vi "二维动态避障简单测试0502(4070双远程版).vi"() -> ()   [LabVIEW 2018]
doc: "Demonstrates the use of the Network Streams functions to send LED status to the myRIO target."
uses:
  <vilib>/addons/zeromq/socket_type.ctl
  <vilib>/ErrorRing/Error Ring.xnode
  <vilib>/vision/NI_Vision_Development_Module.lvlib
  <vilib>/addons/zeromq/zmq_socket.lvclass
  <vilib>/addons/zeromq/zmq_context.lvclass
  <vilib>/addons/zeromq/zeromq.lvlib
panel:
  out "c2":ext
  out "c1":ext
  out "next_relative_desired_point_y":ext
  out "next_relative_desired_point_x":ext
  in  "簇 14":cluster{"c1":ext, "c2":ext}={"c1"=100000.0, "c2"=100000.0}
  out "relative_real_y_color 2":dbl=2.0
  out "relative_real_x_color 2":dbl=2.0
  in  "簇 13":T1={"relative_real_x_color"=100000.0, "relative_real_y_color"=1.0, "t"=1.0}
  out "u(t)_y":ext
  out "u(t)_x":ext
  out "relative_real_y_color":ext
  out "relative_real_x_color":ext
  in  "中心轨迹":bool
  in  "打开彩色点轨迹":bool
  out "relative_real_y_color":ext
  out "relative_real_x_color":ext
  out "彩色轨迹":T2(plugin-control)
  out "end_point_y":ext
  out "end_point_x":ext
  out "cy":ext
  out "cx":ext
  out "c":ext
  in  "簇 10":T3={"c"=100000.0, "cx"=100000.0, "cy"=100000.0, "start_point_x"=100000.0, "start_point_y"=100000.0}
  out "输出簇":T4
  in  "簇 9":T4={"a"=[], "b"=1.0, "a2"=[], "left1"=1.0, "top1"=1.0, "left2"=1.0, "top2"=1.0, "delta1"=1.0, "delta2"=1.0}
  in  "delta2":dbl=130.0
  out "bottom2":dbl
  out "right2":dbl
  out "top2":dbl
  out "left2":dbl
  in  "delta1":dbl=130.0
  out "bottom1":dbl
  out "right1":dbl
  out "top1":dbl
  out "left1":dbl
  out "delta_pr":dbl
  out "delta_dr":dbl
  in  "k2":dbl=-0.3
  in  "K1":dbl=0.3
  in  "Operation":T5(ring)=enum."Erode"
  out "old_real_relative_point_y":dbl
  out "old_real_relative_point_x":dbl
  out "real_relative_start_point_y":dbl
  out "real_relative_start_point_x":dbl
  out "Bounding Box.Y Top 2":i32
  out "Bounding Box.X Left 2":i32
  out "Ki part":dbl
  out "Kd part":dbl
  out "Kp part":dbl
  out "Ki part":dbl
  out "Kd part":dbl
  out "Kp part":dbl
  in  "Ki":dbl=0.004
  in  "Kd":dbl=1e-05
  in  "Kp":dbl=0.013
  in  "Ki":dbl=0.0035
  in  "Kd":dbl=1e-05
  in  "Kp":dbl=0.013
  out "添加的数组":dbl[](array[numeric])
  out "desired_relative_point_y":dbl=820.0
  out "desired_relative_point_x":dbl=730.0
  out "MLP_pr":dbl=20.0
  out "MLP_dr":dbl=8.0
  out "error_relative_point_y":dbl
  out "error_relative_point_x":dbl
  out "real_relative_end_point_y":dbl
  out "real_relative_end_point_x":dbl
  out "magnet_input_pr":dbl
  out "magnet_input_dr":dbl
  in  "打开仅尖端轨迹":bool
  out "仅尖端轨迹":T2(plugin-control)
  out "Bounding Box.Y Top":i32
  out "Bounding Box.X Left":i32
  out "curve_min_y":dbl
  out "curve_min_x":dbl
  out "curve_max_y":dbl
  out "curve_max_x":dbl
  out "relative_end_point_y":dbl
  out "relative_end_point_x":dbl
  out "delta_y":dbl
  out "delta_x":dbl
  out "pr":dbl=-28.0
  out "tan(v)":dbl
  out "delta_velocity":dbl format="%#_10g"
  out "delta_time":dbl
  out "now time":timestamp[](array[timestamp])
  out "prev time":timestamp[](array[timestamp])
  out "delta_distance":dbl
  out "prev_end_point_y":dbl
  out "prev_end_point_x":dbl
  out "now_end_point_y":dbl
  out "now_end_point_x":dbl
  out "prev_end_point_y":dbl[](array[numeric])
  out "prev_end_point_x":dbl[](array[numeric])
  out "dr":dbl=120.0
  in  "Ar":sgl=11.0
  out "all parameters":dbl[][](array[numeric])
  out "direction angle":sgl[](array[numeric])
  out "dr":sgl
  out "strength":dbl[](array[numeric])
  out "场强":dbl
  out "end_point_y":T6
  out "end_point_x":dbl[](array[numeric])
  out "start_point_y":dbl[](array[numeric])
  out "start_point_x":dbl[](array[numeric])
  out "T":i32[](array[numeric])
  out "c":dbl[](array[numeric])
  out "b":dbl[](array[numeric])
  out "a\na":dbl[](array[numeric])
  out "c":dbl
  out "b":dbl
  out "a":dbl
  out "Angles (deg)":sgl[](array[numeric]) format="%.2f"
  in  "wr":sgl
  in  "打开轨迹":bool
  out "中心轨迹和尖端轨迹":T2(plugin-control)
  out "end_y":dbl
  out "end_x":dbl
  out "start_y":dbl
  out "start_x":dbl
  out "Image Pixels (U8)":u8[][](array[numeric])
  in  "Poly":dbl
  out "中心轨迹":T2(plugin-control)
  in  "保存按钮":bool
  out "Object Center":cluster{"X":sgl, "Y":sgl}
  out "黑白图":T2(plugin-control)
  in  "Number of Erosion":i32=5
  in  "Settings":T7={"Objects"=1, "Threshold"=128, "Reject Border"=FALSE, "Fill Holes"=FALSE, "Min Object Size"=TRUE, "Min Size"=1200, "Max Object Size"=FALSE, "Max Size"=100, "Show Search Area"=TRUE, "Show Center"=TRUE, "Show Bounding Box"=TRUE} {"Objects" items=["Bright Objects", "Dark Objects"]; "Threshold" min=1 max=999999999 step=1; "Max Size" min=1 max=999999999 step=1; "Min Size" min=1 max=999999999 step=1}
  out "Objects":T8(array[cluster]) {"Aspect Ratio" format="%.2f"; "Orientation" format="%.2f"; "Area" format="%.2f"; "Object Center"."Y" format="%.2f"; "Object Center"."X" format="%.2f"}
  in  "Search Rect (entire image)":T9={"Left"=350, "Top"=100, "Right"=1020, "Bottom"=1030, "Rotation"=0.0} {"Rotation" format="%.2f"; "Left" scale=0.0..1024.0; "Right" scale=0.0..1024.0}
  in  "Range":cluster{"Lower value":sgl, "Upper value":sgl}={"Lower value"=177.0, "Upper value"=255.0} {"Upper value" format="%.2f"; "Lower value" format="%.2f"}
  out "原图":T2(plugin-control)
  in  "停止":bool
  out "T":i32
  out "T":i32
  in  "磁场变换":bool=TRUE
  in  "Pause":bool
  out "Array":ext[](array[numeric])
  in  "Parameter Settings":T10(tab)=enum."Rotating Field" caption="Field Types"
  in  "Ag":dbl
  in  "dg":dbl
  in  "pg":dbl
  in  "fg":dbl
  in  "AoOF":dbl
  in  "fo":sgl
  in  "do":sgl
  in  "oo":sgl
  in  "po":sgl
  in  "cc":sgl
  in  "pc":sgl
  in  "wc":sgl
  in  "dc":sgl
  in  "Ac":dbl
  in  "Dis phase step":dbl
  in  "Dis phase frequency (Hz)":dbl
  in  "Dis tumbling frequency (Hz)":dbl
  in  "Dis strength(mT)":dbl
  in  "Swa strength (mT)":dbl
  in  "Swa frequency (Hz)":dbl
  in  "Swa pitch angle (deg)":dbl
  in  "Swa direction angle (deg)":dbl
  in  "Swa ratio":dbl=1.0
  in  "Pitch Angle (rotating around Constant, deg)":dbl
  in  "Ratio (A/C)":sgl
  in  "Direction Angle (deg)":sgl
  in  "Pitch Angle (rotating around Origin, deg)":sgl
  in  "Frequency (Hz)":sgl
  in  "Strength (mT)":dbl
  in  "Ar 2":dbl caption="Ar"
  in  "ratio":sgl
  in  "pr  2":sgl
  in  "dr  2":sgl
  in  "wr  2":sgl
  in  "p_x":sgl
  out "Numeric 5":i32
  in  "Stop":bool
  out "error out":errorcluster
  in  "Target IP Address":string="172.22.11.2"
  # "Overview: Magnetic field calculation, and send parameters to myRIO\nInstructions:\n1. Verify the value of Target IP Address. Set Visa resource name.\n2. Ensure RT Main.vi is already running. \n3. Run this VI. Set parameters of magnetic field."
  # "Strength (mT)"
  # "Frequency (Hz)"
  # "Pitch Angle (deg)"
  # "Direction Angle (deg)"
  # "Strength (mT)"
  # "Pitch Angle (deg)"
  # "Direction Angle (deg)"
  # "Frequency (Hz)"
  # "Strength (mT)"
  # "Oscilation Frequency (Hz)"
  # "Oscilation Angle (deg)"
  # "Pitch Angle (deg)"
  # "Direction Angle (deg)"
  # "Strength (mT)"
  # "Frequency (Hz)"
  # "Pitch Angle (deg)"
  # "Direction Angle (deg)"
  # "Conical Angle (deg)"
  # "Strength (mT)"
  # "Tumbling Frequency (Hz)"
  # "Phase Frequency (Hz)"
  # "Phase Step"
  # "Strength (mT)"
  # "Frequency (Hz)"
  # "Pitch Angle (deg)"
  # "Direction Angle (deg)"
  # "Ratio"
  # "Strength (mT)"
  # "Frequency (Hz)"
  # "Ratio (A/C)"
  # "Direction Angle (deg)"
  # "Pitch Angle (rotating around Origin, deg)"
  # "Pitch Angle (rotating around Constant, deg)"
  # "Strength (mT)"
  # "Frequency (Hz)"
  # "Pitch Angle Y (deg)"
  # "Pitch Angle X (deg)"
  # "Direction Angle (deg)"
  # "ratio (l/s)"
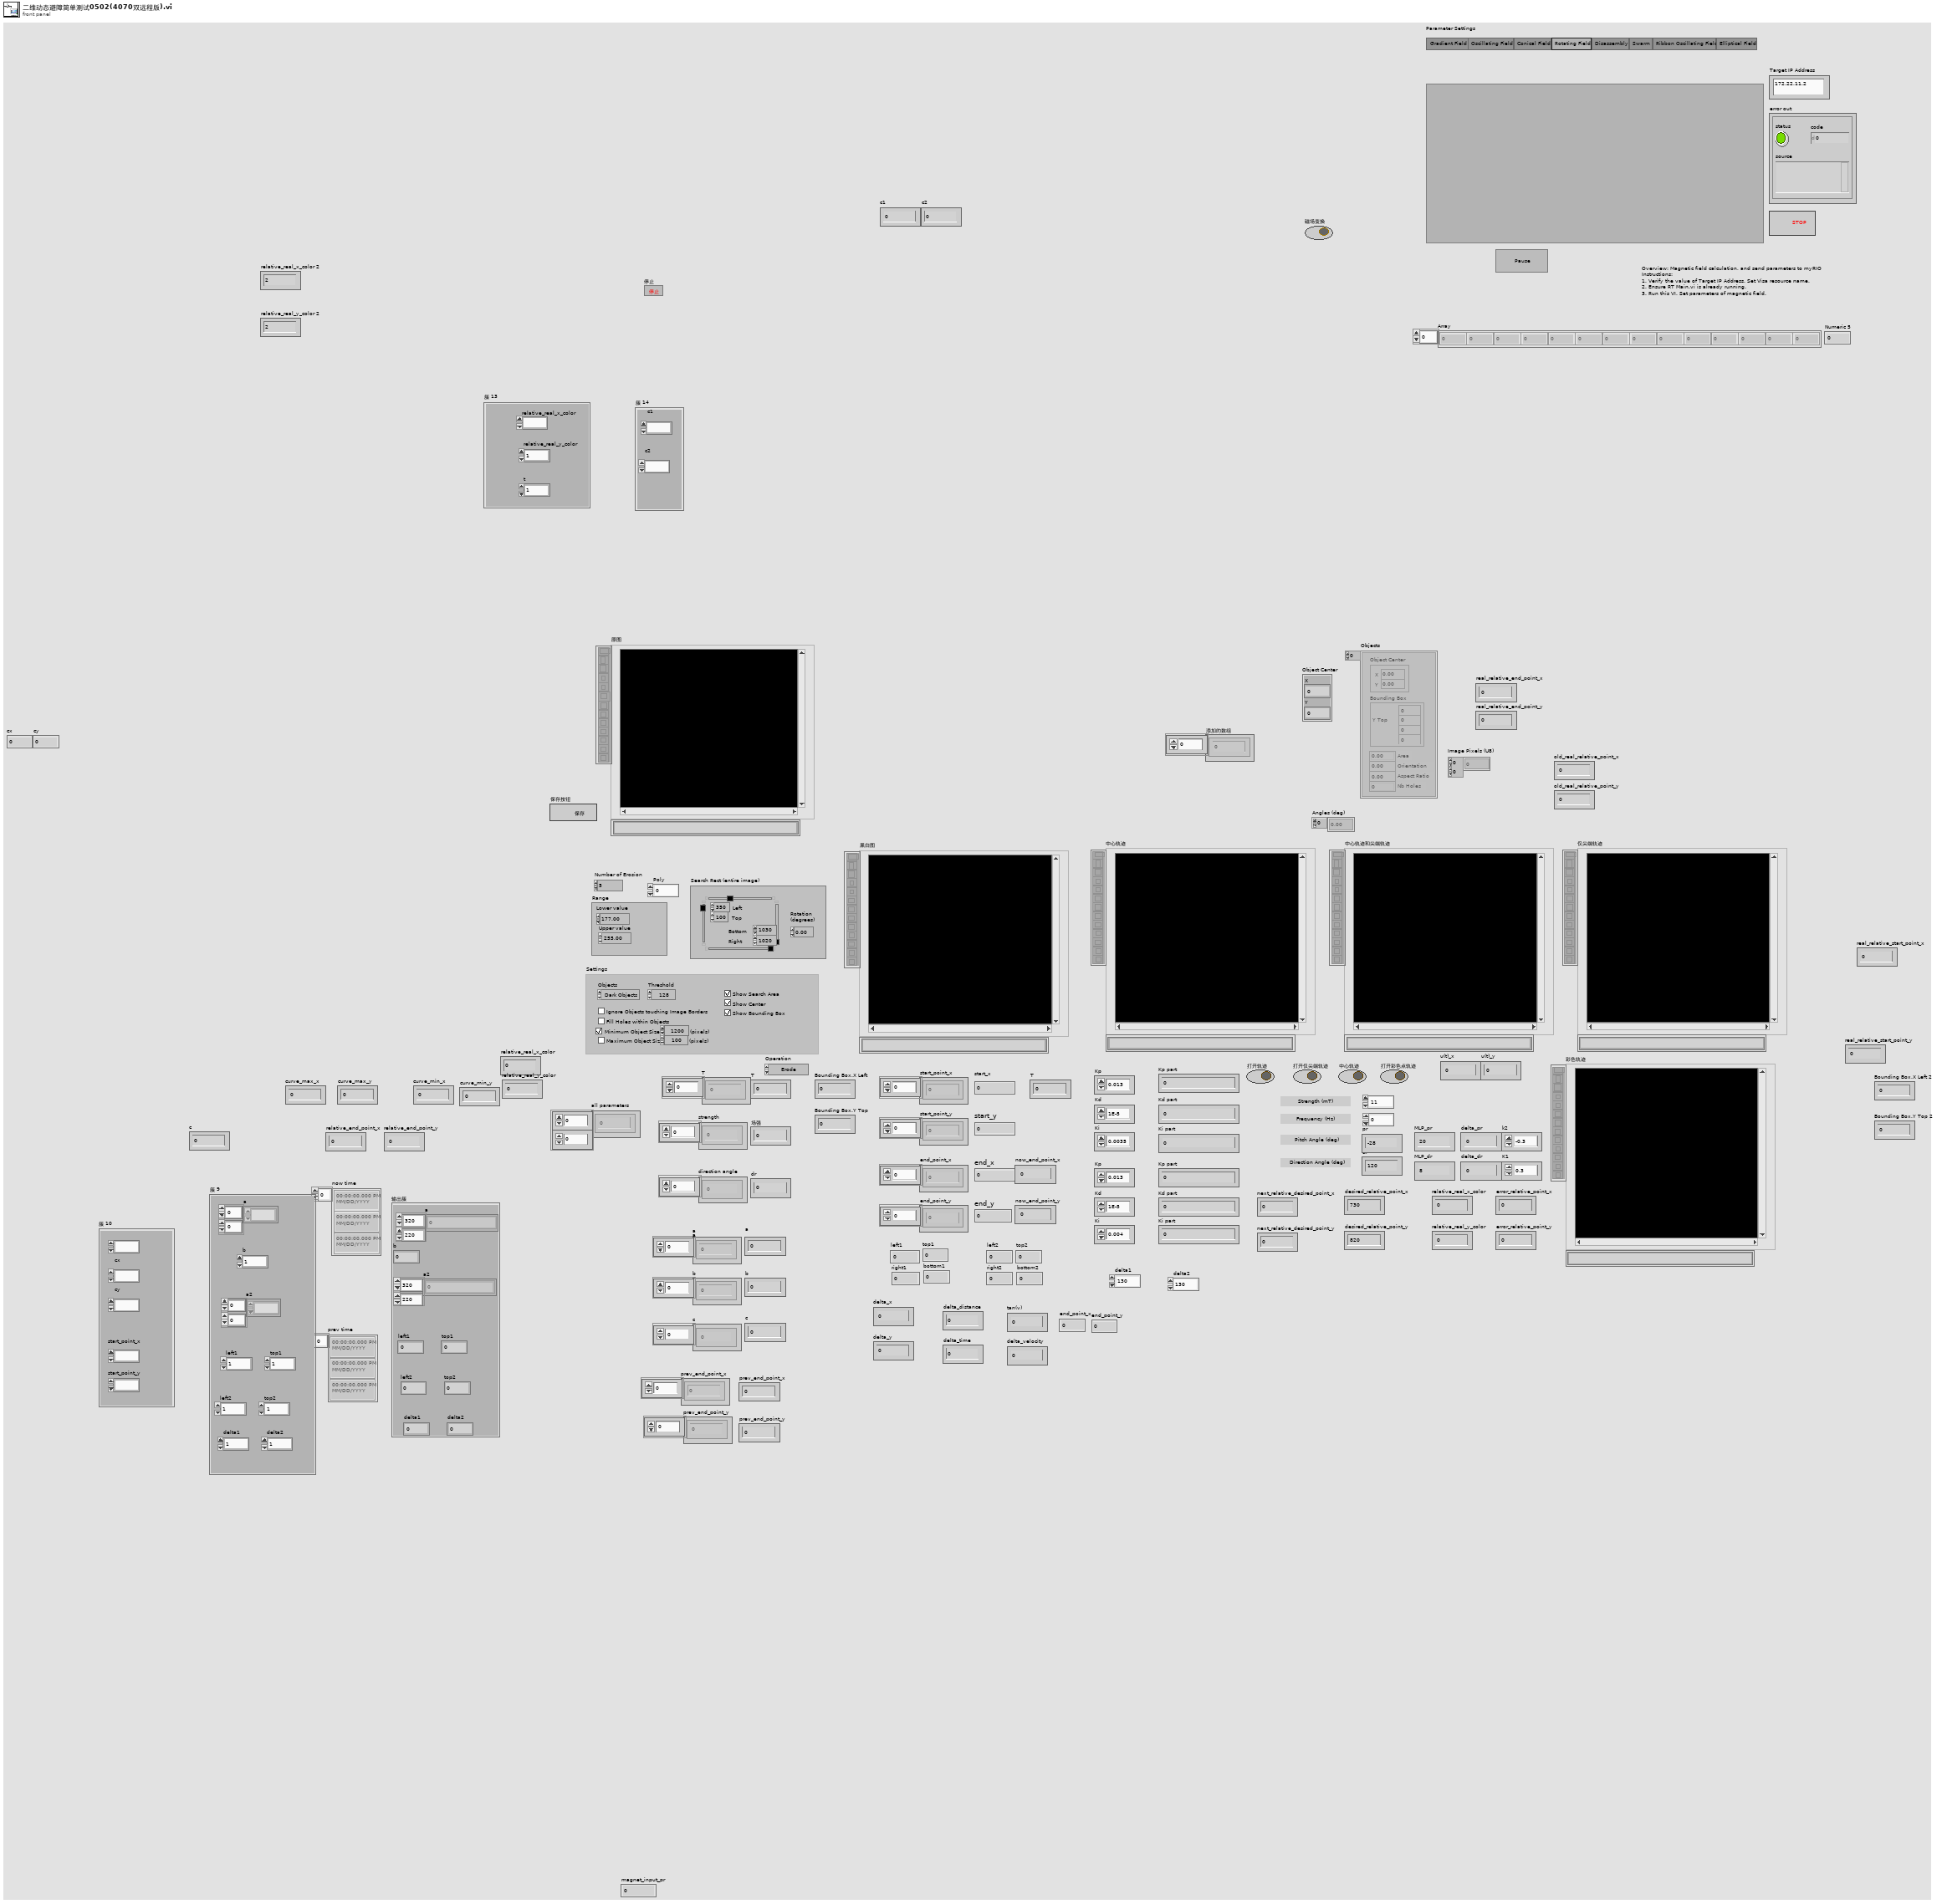
[diagram p1: front panel]
types:
  T1 = cluster{"relative_real_x_color":ext, "relative_real_y_color":dbl, "t":dbl}
  T2 = typedef "IMAQ Image.ctl" = refnum<image>
  T3 = cluster{"c":ext, "cx":ext, "cy":ext, "start_point_x":ext, "start_point_y":ext}
  T4 = cluster{"a":ext[][], "b":dbl, "a2":ext[][], "left1":dbl, "top1":dbl, "left2":dbl, "top2":dbl, "delta1":dbl, "delta2":dbl}
  T5 = enum32{"AutoM", "Close", "Dilate", "Erode", "Gradient", "Gradient in", "Gradient out", "HitMiss", "Open", "PClose", "POpen", "Thick", "Thin"}
  T6 = typedef "控件 3.ctl" = dbl[]
  T7 = cluster{"Objects":u16, "Threshold":i32, "Reject Border":bool, "Fill Holes":bool, "Min Object Size":bool, "Min Size":i32, "Max Object Size":bool, "Max Size":i32, "Show Search Area":bool, "Show Center":bool, "Show Bounding Box":bool}
  T8 = cluster{"Object Center":cluster{"X":sgl, "Y":sgl}, "Bounding Box":cluster{"X Left":i32, "Y Top":i32, "X Right":i32, "Y Bottom":i32}, "Area":sgl, "Orientation":sgl, "Aspect Ratio":sgl, "Nb Holes":i32}[]
  T9 = typedef "IMAQ Rectangle" = cluster{"Left":i32, "Top":i32, "Right":i32, "Bottom":i32, "Rotation":dbl}
  T10 = enum32{"Gradient Field ", "Oscillating Field", "Conical Field", "Rotating Field", "Disassembly", "Swarm", "Ribbon Oscillating Field", "Elliptical Field"}
  T11 = typedef "zeromq.lvlib/socket_type.ctl" = enum8{"ZMQ_PAIR", "ZMQ_PUB", "ZMQ_SUB", "ZMQ_REQ", "ZMQ_REP", "ZMQ_DEALER", "ZMQ_ROUTER", "ZMQ_PULL", "ZMQ_PUSH", "ZMQ_XPUB", "ZMQ_XSUB", "ZMQ_STREAM", "ZMQ_SERVER", "ZMQ_CLIENT", "ZMQ_RADIO", "ZMQ_DISH", "ZMQ_GATHER", "ZMQ_SCATTER", "ZMQ_DGRAM"}
  T12 = typedef "Image Type" = u32
  T13 = cluster{"Object Center":cluster{"X":sgl, "Y":sgl}, "Bounding Box":cluster{"X Left":i32, "Y Top":i32, "X Right":i32, "Y Bottom":i32}, "Area":sgl, "Orientation":sgl, "Aspect Ratio":sgl, "Nb Holes":i32}
  T14 = cluster{"X Left":i32, "Y Top":i32, "X Right":i32, "Y Bottom":i32, "Rotation":dbl}
  T15 = typedef "ROI Descriptor" = cluster{"Global Rectangle":i32[], "Contours":cluster{"ID":enum32{"External", "Internal"}, "Type":u32, "Coordinates":i32[]}[]}
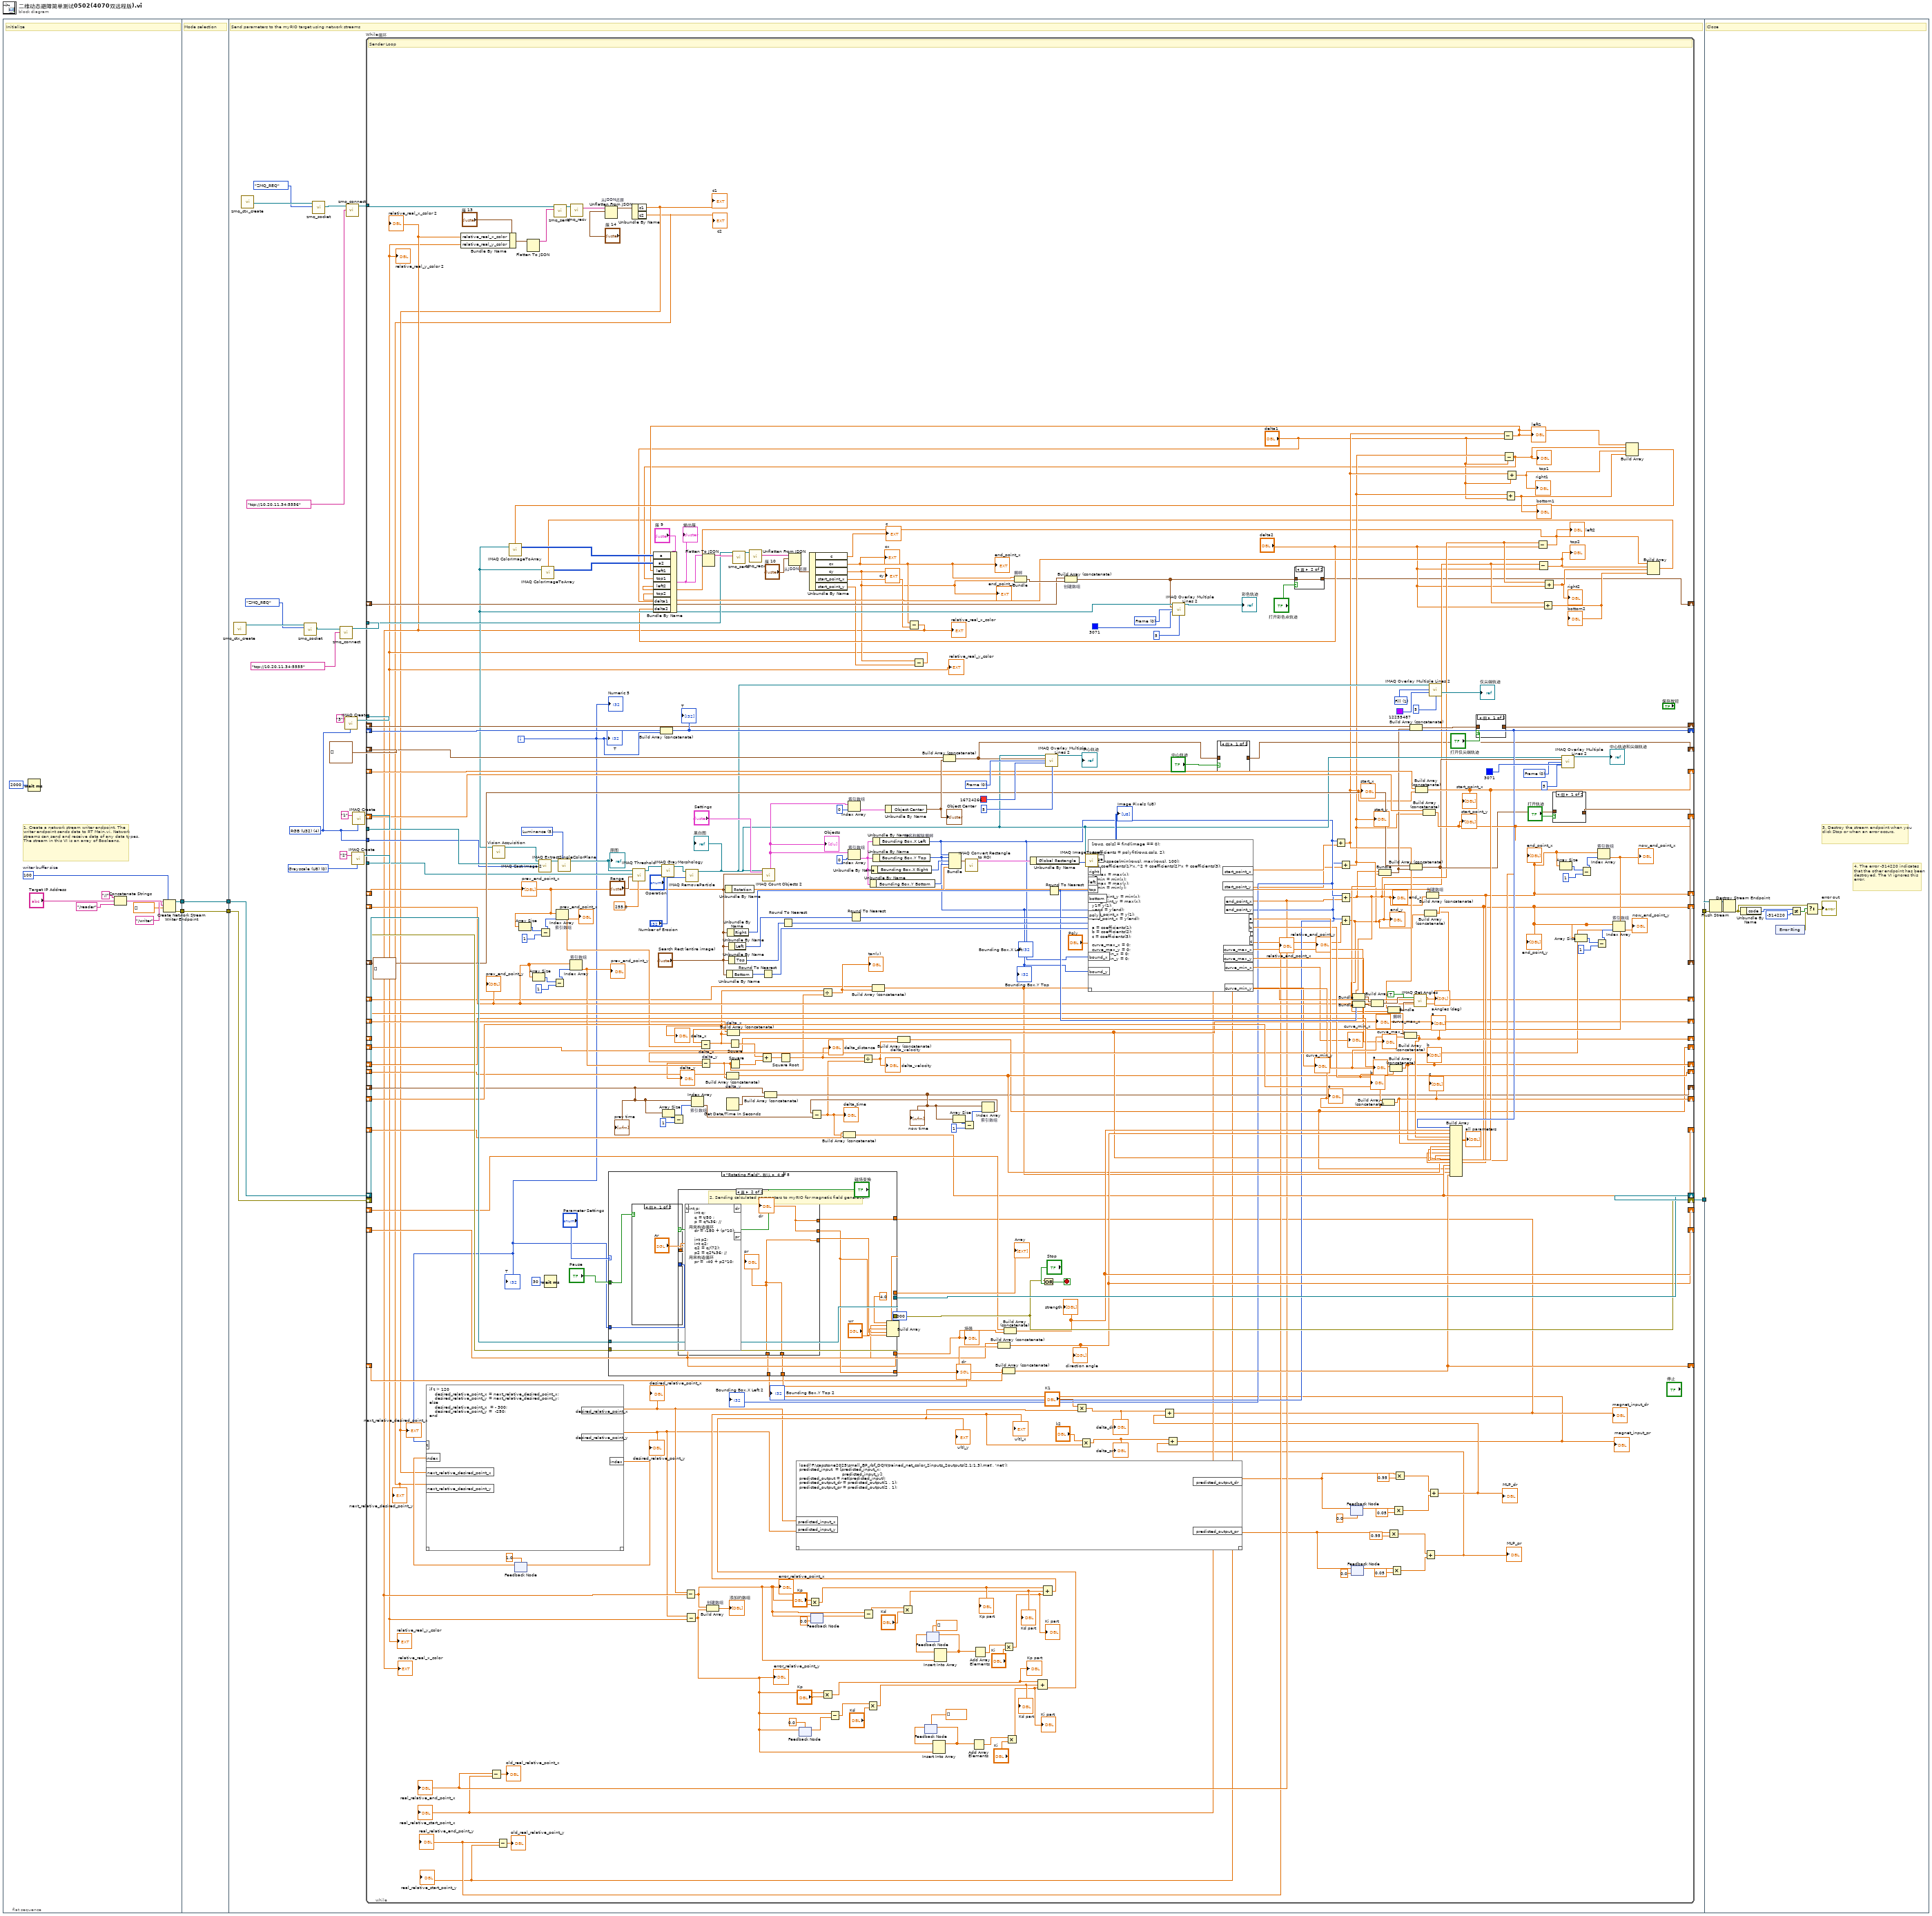
[diagram p0: block diagram]
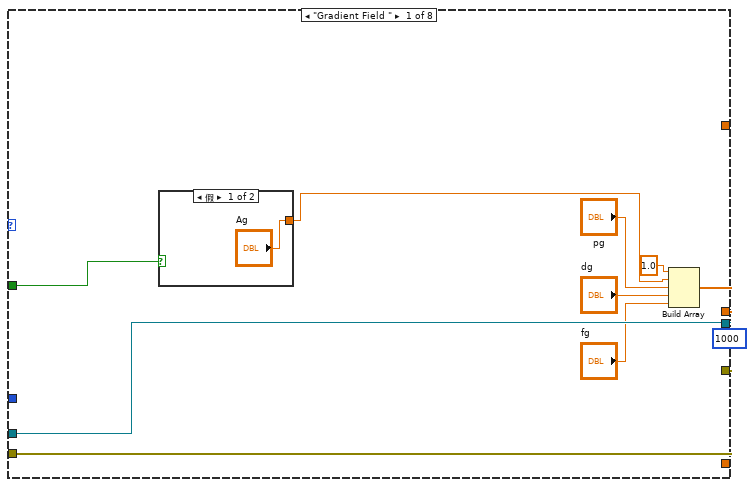
[diagram p6: hidden frame]
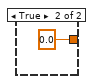
[diagram p7: hidden frame]
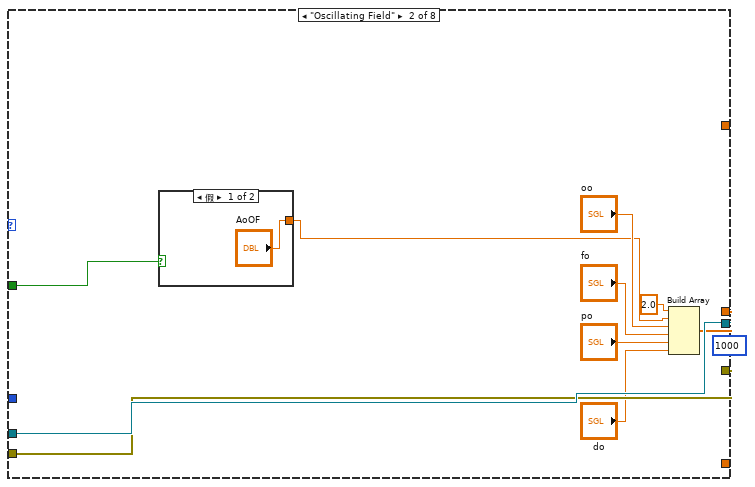
[diagram p8: hidden frame]
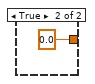
[diagram p9: hidden frame]
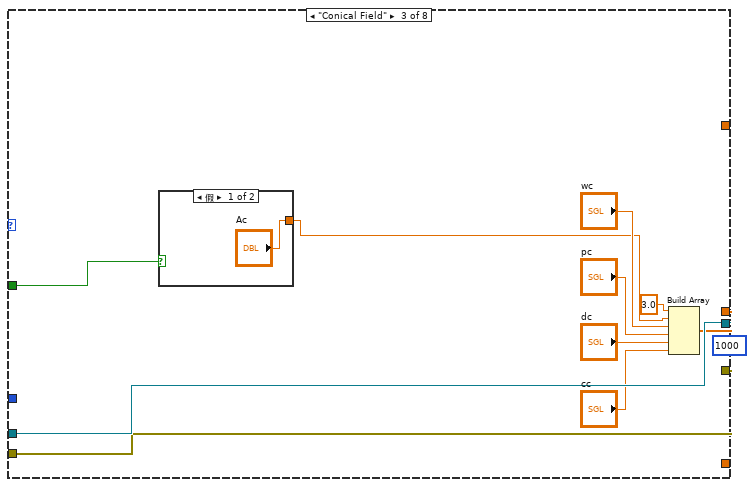
[diagram p10: hidden frame]
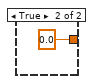
[diagram p11: hidden frame]
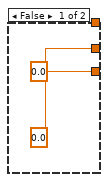
[diagram p12: hidden frame]
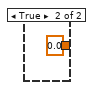
[diagram p13: hidden frame]
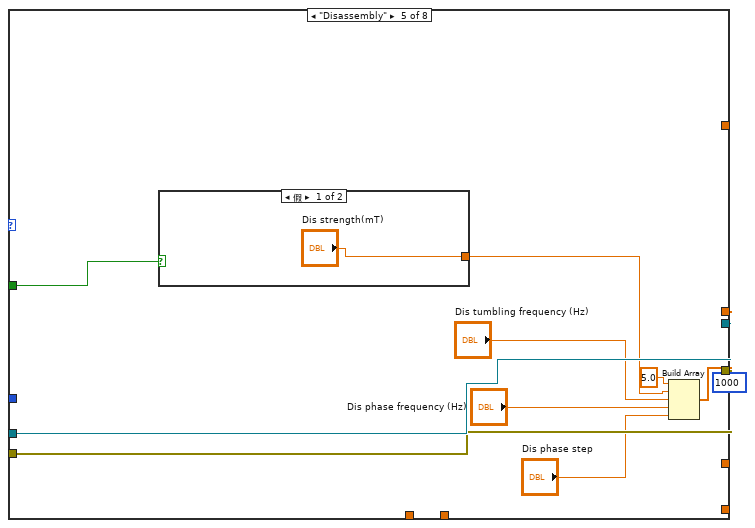
[diagram p14: hidden frame]
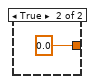
[diagram p15: hidden frame]
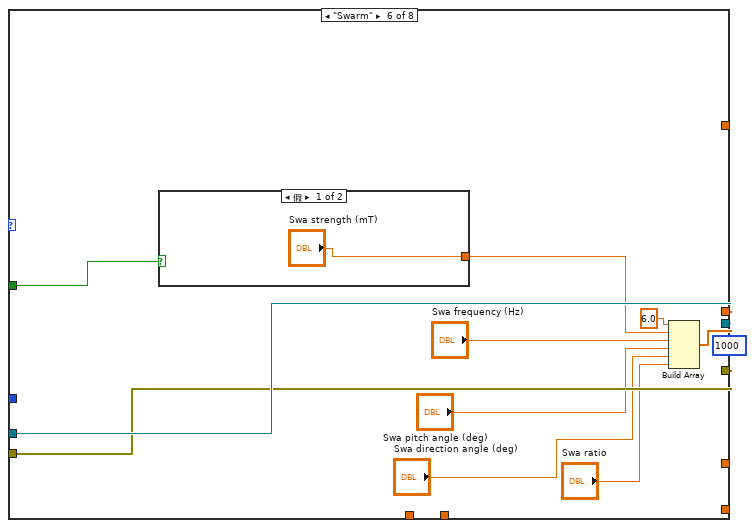
[diagram p16: hidden frame]
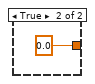
[diagram p17: hidden frame]
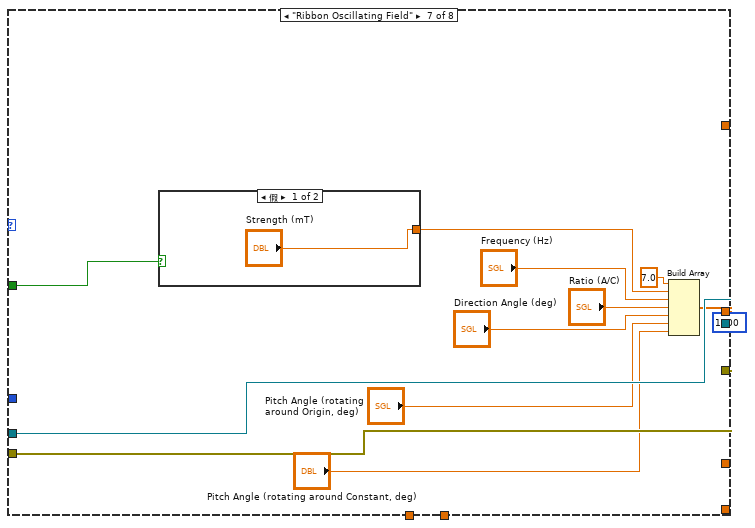
[diagram p18: hidden frame]
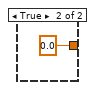
[diagram p19: hidden frame]
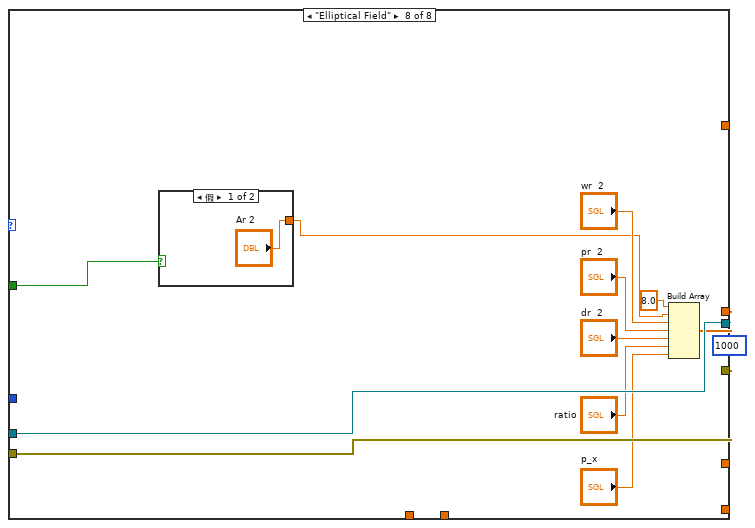
[diagram p20: hidden frame]
diagram:
  n1 = flat-sequence {
    tunnel: [w11] -> w2
    tunnel: [w10] -> w1
    tunnel: [w18] -> w4
    tunnel: [w17] -> w3
    tunnel: w1 -> [w17]
    tunnel: w2 -> [w18]
    tunnel: [w40] -> w6
    tunnel: w4 -> [w42]
    tunnel: [w39] -> w5
    tunnel: w3 -> [w41]
    tunnel: w6 -> [w462]
    tunnel: w5 -> [w459]
    frame #0 {
      w9 = 100  # writer buffer size
      # "1. Create a network stream writer endpoint. The writer endpoint sends data to RT Main.vi. Network streams can send and receive data of any data types. The stream in this VI is an array of Booleans."
      # "Initialize"
      n2 = Wait (ms)(milliseconds to wait=2000) -> ()  [unwired: 1 out]
      n3 = Concatenate Strings("//", "Target IP Address", "/reader") -> (w16:string)
      n4 = Create Network Stream Writer Endpoint(7:w9, 9:dbl[] [], 10:w16, 11:"/writer" ("reader name")) -> (0:w10:errorcluster, 3:w11:refnum<k21>)  [unwired: 3 in]
    }
    frame #1 {
      # "Mode selection"
    }
    frame #2 {
      w36 = T12 0 items=["Grayscale (U8)", "Grayscale (I16)", "Grayscale (SGL)", "Complex (CSG)", "RGB (U32)", "HSL (U32)", "RGB (U64)", "Grayscale (U16)"] ("Image Type")
      w29 = T12 4 items=["Grayscale (U8)", "Grayscale (I16)", "Grayscale (SGL)", "Complex (CSG)", "RGB (U32)", "HSL (U32)", "RGB (U64)", "Grayscale (U16)"] ("Image Type")
      # "Send parameters to the myRIO target using network streams"
      n5 = call <vilib>:"zmq_ctx_create.vi"() -> ("context out"=w27:refnum<class "zmq_context.lvclass">)  [unwired: 4 in, 1 out]
      n6 = call <vilib>:"zmq_ctx_create.vi"() -> ("context out"=w22:refnum<class "zmq_context.lvclass">)  [unwired: 4 in, 1 out]
      n7 = call <vilib>:"zmq_socket.vi"("socket type"=socket_type."ZMQ_REQ", "context in"=w27) -> ("socket out"=w28:refnum<class "zmq_socket.lvclass">)  [unwired: 3 in, 2 out]
      n8 = call <vilib>:"zmq_socket.vi"("socket type"=socket_type."ZMQ_REQ", "context in"=w22) -> ("socket out"=w23:refnum<class "zmq_socket.lvclass">)  [unwired: 3 in, 2 out]
      n9 = call <vilib>:"zmq_connect.vi"("endpoint"="tcp://10.20.11.34:5555", "socket in"=w28) -> ("socket out"=w24:refnum<class "zmq_socket.lvclass">)  [unwired: 2 in, 1 out]
      n10 = call "IMAQ Create"("Image Name"="3", "Image Type"=w29) -> ("New Image"=w32:T2)  [unwired: 3 in, 1 out]
      n11 = call <vilib>:"zmq_connect.vi"("endpoint"="tcp://10.20.11.34:5556", "socket in"=w23) -> ("socket out"=w19:refnum<class "zmq_socket.lvclass">)  [unwired: 2 in, 1 out]
      n12 = call "IMAQ Create"("Image Name"="2", "Image Type"=w36) -> ("New Image"=w34:T2)  [unwired: 3 in, 1 out]
      n13 = call "IMAQ Create"("Image Name"="1", "Image Type"=w29) -> ("New Image"=w35:T2)  [unwired: 3 in, 1 out]
      n14 = while "While循环" {
        shift-right: [w315] -> w39
        shift-left: w41 -> [w317]
        shift-right: [w316] -> w40
        shift-left: w42 -> [w318]
        tunnel: w35 -> [w271]
        tunnel: w34 -> [w270]
        tunnel: w32 -> [_]
        shift-right: [w267] -> _
        shift-left: cluster{"X":dbl, "Y":dbl}[] [] -> [w272]
        shift-right: [w63] -> _
        shift-left: cluster{"X":dbl, "Y":dbl}[] [] -> [w273]
        tunnel: w29 -> [w269]
        shift-right: [w243] -> _
        shift-left: _ -> [w259]
        shift-right: [w238] -> _
        shift-left: _ -> [w257]
        shift-right: [w242] -> _
        shift-left: _ -> [w254]
        shift-right: [w246] -> _
        shift-left: _ -> [w253]
        shift-right: [w241] -> _
        shift-left: _ -> [w252]
        shift-right: [w240] -> _
        shift-left: _ -> [w251]
        shift-right: [w234] -> _
        shift-left: _ -> [w226]
        shift-right: [w230] -> _
        shift-left: _ -> [w222]
        shift-right: [w245] -> _
        shift-left: _ -> [w249]
        shift-right: [w244] -> _
        shift-left: _ -> [w247]
        shift-right: [w211] -> _
        shift-left: _ -> [w213]
        shift-right: [w210] -> _
        shift-left: _ -> [w212]
        shift-right: [w200] -> _
        shift-left: _ -> [w205]
        shift-right: [w197] -> _
        shift-left: _ -> [w198]
        shift-right: [w193] -> _
        shift-left: _ -> [w194]
        shift-right: [w188] -> _
        shift-left: _ -> [w189]
        shift-right: [w180] -> _
        shift-left: _ -> [w181]
        shift-right: [w174] -> _
        shift-left: _ -> [w175]
        shift-right: [w67] -> _
        shift-left: _ -> [w84]
        tunnel: w24 -> [w82]
        tunnel: w19 -> [w52]
        i -> [w51]
        stop <- w311 stop-if-true
        w92 = u32 0 items=["Frame", "Fill"] ("Drawing Mode (Frame)")
        w176 = u32 1 items=["Frame", "Fill"] ("Drawing Mode (Frame)")
        w183 = u32 0 items=["Frame", "Fill"] ("Drawing Mode (Frame)")
        w298 = u32 0 items=["Frame", "Fill"] ("Drawing Mode (Frame)")
        w308 = 5 items=["Red", "Green", "Blue", "Hue", "Saturation", "Luminance", "Value", "Intensity"] ("Color Plane")
        # "2. Sending calculated parameters to myRIO for magnetic field generation."
        # "Sender Loop"
        n15 = call "Vision Acquisition"() -> ("Image Out"=w81:T2)  [unwired: 23 in, 4 out]
        n16 = feedback #1(1.0) -> (w78:dbl)
        n17 = Array Size(array=w226) -> (size(s)=w228:i32)
        n18 = Array Size(array=w222) -> (size(s)=w224:i32)
        n19 = call "IMAQ Cast Image 2"("Image Src"=w81, "Image Dst"=w271, "Image Type"=w269) -> ("Image Dst Out"=w309:T2)  [unwired: 11 in, 1 out]
        n20 = Subtract(x=w228, y=1) -> (x-y=w227:i32)
        n21 = Wait (ms)(milliseconds to wait=u32 30 ("等待时间（毫秒）")) -> ()  [unwired: 1 out]
        n22 = Subtract(x=w224, y=1) -> (x-y=w223:i32)
        n23 = Index Array "索引数组"(array=w226, index=w227) -> (element=w220:dbl)
        "prev_end_point_x" <- w220
        n24 = call "IMAQ ExtractSingleColorPlane"("Color Plane"=w308, "Image Src"=w309) -> ("Image Dst Out"=w307:T2)  [unwired: 8 in, 1 out]
        "原图" <- w307
        n25 = Index Array "索引数组"(array=w222, index=w223) -> (element=w219:dbl)
        "prev_end_point_y" <- w219
        n26 = call "IMAQ Threshold"("Replace Value"=sgl 255.0, "Range"="Range", "Image Dst"=w270, "Image Src"=w307) -> ("Image Dst Out"=w133:T2)  [unwired: 6 in, 1 out]
        n27 = Build Array (concatenate)(w253, w51) -> (w246:i32[])
        "T" <- w246
        n28 = call "IMAQ GrayMorphology"("Operation"="Operation", "Image Src"=w133) -> ("Image Dst Out"=w132:T2)  [unwired: 8 in, 1 out]
        n29 = Array Size(array=w205) -> (size(s)=w208:i32)
        n30 = Subtract(x=w208, y=1) -> (x-y=w207:i32)
        n31 = call "IMAQ RemoveParticle"("Number of Erosion"="Number of Erosion", "Image Src"=w132) -> ("Image Dst Out"=w172:T2)  [unwired: 8 in, 1 out]
        "黑白图" <- w172
        n32 = Index Array "索引数组"(array=w205, index=w207) -> (element=w204:timestamp)
        n33 = Unbundle By Name("Search Rect (entire image)") -> ("Rotation"=w294:dbl)
        n34 = Unbundle By Name("Search Rect (entire image)") -> ("Bottom"=w278:i32)
        n35 = Get Date/Time In Seconds() -> (seconds since 1Jan1904=w209:timestamp)
        n36 = Unbundle By Name("Search Rect (entire image)") -> ("Right"=w282:i32)
        n37 = Unbundle By Name("Search Rect (entire image)") -> ("Left"=w281:i32)
        n38 = Unbundle By Name("Search Rect (entire image)") -> ("Top"=w280:i32)
        n39 = Round To Nearest(number=w278) -> (nearest integer value=w277:i32)
        n40 = call "IMAQ Count Objects 2"("Settings"="Settings", "Search Rect (entire image)"="Search Rect (entire image)", "Image"=w172) -> ("Objects"=w296:T8)  [unwired: 4 in, 4 out]
        "Objects" <- w296
        n41 = Build Array (concatenate)(w205, w209) -> (w200:timestamp[])
        "now time" <- w200
        n42 = Round To Nearest(number=w280) -> (nearest integer value=w279:i32)
        n43 = feedback #2(0.0) -> (w151:ext)
        n44 = feedback #3(0.0) -> (w165:ext)
        n45 = Index Array "索引数组"(array=w296, index=0 ("索引")) -> (element=w301:T13)
        n46 = Index Array "索引数组"(array=w296, index=0 ("索引")) -> (element=w292:T13)
        n47 = Round To Nearest(number=w281) -> (nearest integer value=w275:i32)
        n48 = Unbundle By Name(w292) -> ("Bounding Box.Y Bottom"=w286:i32)
        n49 = Unbundle By Name(w292) -> ("Bounding Box.X Right"=w287:i32)
        n50 = Unbundle By Name "按名称解除捆绑"(w292) -> ("Bounding Box.X Left"=w139:i32)
        "Bounding Box.X Left" <- w139
        "Bounding Box.X Left 2" <- w139
        n51 = Unbundle By Name(w292) -> ("Bounding Box.Y Top"=w138:i32)
        "Bounding Box.Y Top" <- w138
        "Bounding Box.Y Top 2" <- w138
        n52 = Unbundle By Name(w301) -> ("Object Center"=w300:cluster{"X":sgl, "Y":sgl})
        "Object Center" <- w300
        n53 = feedback #4(dbl[] []) -> (w146:dbl[])
        n54 = feedback #5(dbl[] []) -> (w160:dbl[])
        n55 = Build Array (concatenate)(w273, w300) -> (w64:cluster{"X":dbl, "Y":dbl}[])
        n56 = Bundle("X Left"=w139, "Y Top"=w138, "X Right"=w287, "Y Bottom"=w286, "Rotation"=w294) -> (w293:T14)  [unwired: 1 in]
        n57 = Array Size(array=w200) -> (size(s)=w203:i32)
        n58 = Subtract(x=w203, y=1) -> (x-y=w202:i32)
        n59 = call "IMAQ Convert Rectangle to ROI"("Rectangle"=w293) -> ("ROI Descriptor"=w291:T15)  [unwired: 8 in, 1 out]
        n60 = Index Array "索引数组"(array=w200, index=w202) -> (element=w199:timestamp)
        n61 = Subtract(x=w199, y=w204) -> (x-y=w196:dbl)
        "delta_time" <- w196
        n62 = Build Array (concatenate)(w198, w196) -> (w197:dbl[])
        n63 = Unbundle By Name(w291) -> ("Global Rectangle"=w276:i32[])
        n64 = call "IMAQ Overlay Multiple Lines 2"("Image"=w172, "Line End Points"=w64, "Drawing Mode (Frame)"=w298, "Color"=u32 16724266, "Width"=u32 5) -> ("Image Out"=→"中心轨迹":T2)  [unwired: 9 in, 1 out]
        n65 = Round To Nearest(number=w282) -> (nearest integer value=w260:i32)
        n66 = call "IMAQ ImageToArray"("Optional Rectangle"=w276, "Image"=w172) -> ("Image Pixels (U8)"=w288:u8[][])  [unwired: 2 in, 4 out]
        "Image Pixels (U8)" <- w288
        n67 = script code="[rows, cols] = find(image == 0); \n\ncoefficients = polyfit(rows,cols, 2);\n\nx = linspace(min(rows), max(rows), 100); \ny = coefficients(1)*x.^2 + coefficients(2)*x + coefficients(3);\n\nx_max = max(x);\nx_min = min(x);\ny_max = max(y);\ny_min = min(y);\n\nstart_point_y = min(x);\nend_point_y = max(x);\ny1= y(1);\nyend = y(end);\nstart_point_x = y(1);\nend_point_x = y(end);\n\na = coefficients(1);\nb = coefficients(2);\nc = coefficients(3);\n\ncurve_max_x = 0;\ncurve_max_y = 0;\ncurve_min_x = 0;\ncurve_min_y = 0;"("image"=w288, "poly"="Poly", "right"=w260, "left"=w275, "top"=w279, "bottom"=w277, "bound_x"=w139, "bound_y"=w138) -> ("start_point_x"=w136:dbl, "start_point_y"=w134:dbl, "end_point_x"=w137:dbl, "end_point_y"=w135:dbl, "a"=w258:dbl, "b"=w256:dbl, "c"=w255:dbl, "curve_max_x"=→"curve_max_x":dbl, "curve_max_y"=→"curve_max_y":dbl, "curve_min_x"=→"curve_min_x":dbl, "curve_min_y"=→"curve_min_y":dbl)  [unwired: 1 in, 1 out]
        "a" <- w258
        "b" <- w256
        "c" <- w255
        "relative_end_point_x" <- w137
        "relative_end_point_y" <- w135
        "real_relative_end_point_x" <- w137
        "real_relative_end_point_y" <- w135
        "real_relative_start_point_x" <- w136
        "real_relative_start_point_y" <- w134
        n68 = Subtract(x=w137, y=w136) -> (x-y=→"old_real_relative_point_x":dbl)
        n69 = Subtract(x=w135, y=w134) -> (x-y=→"old_real_relative_point_y":dbl)
        n70 = case shown="假" "中心轨迹" {
          tunnel: w64 -> [_ w320]
          tunnel: [_ w320] -> w63
          frame False {
          }
          frame True {
          }
        }
        n71 = Add(x=w139, y=w136) -> (x+y=w106:dbl)
        "start_x" <- w106
        n72 = Add(x=w138, y=w134) -> (x+y=w105:dbl)
        "start_y" <- w105
        n73 = Add(x=w139, y=w137) -> (x+y=w104:dbl)
        "end_x" <- w104
        n74 = Add(x=w138, y=w135) -> (x+y=w103:dbl)
        "end_y" <- w103
        n75 = feedback #6(0.0) -> (w128:dbl)
        n76 = feedback #7(0.0) -> (w120:dbl)
        n77 = Bundle(w104, w103) -> (w264:cluster{dbl, dbl})  [unwired: 1 in]
        n78 = Bundle(w260, w105) -> (w263:cluster{i32, dbl})  [unwired: 1 in]
        n79 = Build Array(w264, w263) -> (w262:cluster{dbl, dbl}[])
        n80 = Bundle(w104, w103) -> (w170:cluster{dbl, dbl})  [unwired: 1 in]
        n81 = Build Array (concatenate)(w254, w255) -> (w242:dbl[])
        "c" <- w242
        n82 = Bundle "捆绑"(w106, w105) -> (w265:cluster{dbl, dbl})  [unwired: 1 in]
        n83 = Build Array (concatenate)(w257, w256) -> (w238:dbl[])
        "b" <- w238
        n84 = Multiply(x=w120, y=0.05) -> (x*y=w117:dbl)
        n85 = Multiply(x=w128, y=0.05) -> (x*y=w124:dbl)
        n86 = Build Array (concatenate)(w259, w258) -> (w243:dbl[])
        "a\na" <- w243
        n87 = Build Array (concatenate)(w272, w170) -> (w171:cluster{"X":dbl, "Y":dbl}[])
        n88 = Build Array (concatenate)(w175, w170) -> (w169:cluster{dbl, dbl}[])
        n89 = call "IMAQ Get Angles"("Vertex"=w265, "Points"=w262, "Use Vertex (No)"=TRUE) -> ("Angles (deg)"=→"Angles (deg)":sgl[])  [unwired: 2 in, 2 out]
        n90 = Build Array (concatenate)(w252, w106) -> (w241:dbl[])
        "start_point_x" <- w241
        n91 = Build Array (concatenate)(w251, w105) -> (w240:dbl[])
        "start_point_y" <- w240
        n92 = Build Array (concatenate)(w222, w103) -> (w230:dbl[])
        "end_point_y" <- w230
        n93 = Build Array (concatenate) "创建数组"(w226, w104) -> (w234:dbl[])
        "end_point_x" <- w234
        n94 = call "IMAQ Overlay Multiple Lines 2"("Image"=w172, "Drawing Mode (Frame)"=w176, "Color"=u32 12255487, "Width"=u32 5) -> ("Image Out"=→"仅尖端轨迹":T2)  [unwired: 10 in, 1 out]
        n95 = case shown="假" "打开仅尖端轨迹" {
          tunnel: [_ w322] -> w174
          tunnel: w169 -> [_ w322]
          frame False {
          }
          frame True {
          }
        }
        n96 = Subtract(x=w106, y="delta1") -> (x-y=w87:dbl)
        "left1" <- w87
        n97 = Subtract(x=w105, y="delta1") -> (x-y=w86:dbl)
        "top1" <- w86
        n98 = Add(x=w105, y="delta1") -> (x+y=w107:dbl)
        "bottom1" <- w107
        n99 = Add(x=w106, y="delta1") -> (x+y=w108:dbl)
        "right1" <- w108
        n100 = Subtract(x=w104, y="delta2") -> (x-y=w85:dbl)
        "left2" <- w85
        n101 = Subtract(x=w103, y="delta2") -> (x-y=w83:dbl)
        "top2" <- w83
        n102 = Add(x=w103, y="delta2") -> (x+y=w109:dbl)
        "bottom2" <- w109
        n103 = Add(x=w104, y="delta2") -> (x+y=w110:dbl)
        "right2" <- w110
        n104 = case shown="假" "打开轨迹" {
          tunnel: [_ w323] -> w267
          tunnel: w171 -> [_ w323]
          frame False {
          }
          frame True {
          }
        }
        n105 = Array Size(array=w234) -> (size(s)=w236:i32)
        n106 = call "IMAQ Overlay Multiple Lines 2"("Image"=w172, "Line End Points"=w171, "Drawing Mode (Frame)"=w183, "Color"=u32 3071, "Width"=u32 5) -> ("Image Out"=→"中心轨迹和尖端轨迹":T2)  [unwired: 9 in, 1 out]
        n107 = Array Size(array=w230) -> (size(s)=w232:i32)
        n108 = Subtract(x=w236, y=1) -> (x-y=w235:i32)
        n109 = Subtract(x=w232, y=1) -> (x-y=w231:i32)
        n110 = Index Array "索引数组"(array=w234, index=w235) -> (element=w221:dbl)
        "now_end_point_x" <- w221
        n111 = Subtract "delta_x"(x=w221, y=w220) -> (x-y=w192:dbl)
        "delta_x" <- w192
        n112 = Build Array (concatenate) "delta_x"(w213, w192) -> (w211:dbl[])
        n113 = Square(x=w192) -> (x^2=w217:dbl)
        n114 = Index Array "索引数组"(array=w230, index=w231) -> (element=w218:dbl)
        "now_end_point_y" <- w218
        n115 = Subtract "delta_y"(x=w218, y=w219) -> (x-y=w191:dbl)
        "delta_y" <- w191
        n116 = Build Array (concatenate) "delta_y"(w212, w191) -> (w210:dbl[])
        n117 = Square(x=w191) -> (x^2=w216:dbl)
        n118 = Add(x=w217, y=w216) -> (x+y=w215:dbl)
        n119 = Square Root(x=w215) -> (sqrt(x)=w214:dbl)
        "delta_distance" <- w214
        n120 = Divide(x=w192, y=w191) -> (x/y=w190:dbl)
        "tan(v)" <- w190
        n121 = Divide(x=w214, y=w196) -> (x/y=w195:dbl)
        "delta_velocity" <- w195
        n122 = Build Array (concatenate)(w189, w190) -> (w188:dbl[])
        n123 = Build Array (concatenate) "delta_velocity"(w194, w195) -> (w193:dbl[])
        n124 = Build Array(w87, w86, w108, w107) -> (w102:dbl[])
        n125 = call "IMAQ ColorImageToArray"("Optional Rectangle"=w102, "Image"=w81) -> ("Image Pixels (U32)"=w89:u32[][])  [unwired: 2 in, 2 out]
        n126 = Build Array(w85, w83, w110, w109) -> (w60:dbl[])
        n127 = call "IMAQ ColorImageToArray"("Optional Rectangle"=w60, "Image"=w81) -> ("Image Pixels (U32)"=w88:u32[][])  [unwired: 2 in, 2 out]
        n128 = Bundle By Name(cluster="簇 9", "a"=w89, "a2"=w88, "left1"=w87, "top1"=w86, "left2"=w85, "top2"=w83, "delta1"="delta1", "delta2"="delta2") -> (w95:T4)
        "输出簇" <- w95
        n129 = Flatten To JSON(anything=w95) -> (JSON string=w94:string)  [unwired: 2 in, 1 out]
        n130 = call <vilib>:"zmq_send.vi"("data"=w94, "socket in"=w82) -> ("socket out"=w99:refnum<class "zmq_socket.lvclass">)  [unwired: 5 in, 1 out]
        n131 = call <vilib>:"zmq_recv.vi"("socket in"=w99) -> ("data"=w100:string)  [unwired: 4 in, 4 out]
        n132 = Unflatten From JSON "从JSON还原"(JSON string=w100, type and defaults="簇 10") -> (value=w97:T3)  [unwired: 5 in, 1 out]
        n133 = Unbundle By Name(w97) -> ("c"=→"c":ext, "cx"=w72:ext, "cy"=w70:ext, "start_point_x"=w71:ext, "start_point_y"=w69:ext)
        "cx" <- w72
        "cy" <- w70
        "end_point_x" <- w72
        "end_point_y" <- w70
        n134 = Subtract(x=w72, y=w71) -> (x-y=w50:ext)
        "relative_real_x_color" <- w50
        "relative_real_x_color" <- w50
        "relative_real_x_color 2" <- w50
        n135 = Subtract(x=w70, y=w69) -> (x-y=w49:ext)
        "relative_real_y_color" <- w49
        "relative_real_y_color" <- w49
        "relative_real_y_color 2" <- w49
        n136 = Bundle By Name(cluster="簇 13", "relative_real_x_color"=w50, "relative_real_y_color"=w49) -> (w58:T1)
        n137 = Flatten To JSON(anything=w58) -> (JSON string=w53:string)  [unwired: 2 in, 1 out]
        n138 = call <vilib>:"zmq_send.vi"("data"=w53, "socket in"=w52) -> ("socket out"=w56:refnum<class "zmq_socket.lvclass">)  [unwired: 5 in, 1 out]
        n139 = call <vilib>:"zmq_recv.vi"("socket in"=w56) -> ("data"=w57:string)  [unwired: 4 in, 4 out]
        n140 = Unflatten From JSON "从JSON还原"(JSON string=w57, type and defaults="簇 14") -> (value=w54:cluster{"c1":ext, "c2":ext})  [unwired: 5 in, 1 out]
        n141 = Unbundle By Name(w54) -> ("c1"=w48:ext, "c2"=w47:ext)
        "next_relative_desired_point_x" <- w48
        "next_relative_desired_point_y" <- w47
        "c1" <- w48
        "c2" <- w47
        n142 = script code="if t > 120\n    desired_relative_point_x = next_relative_desired_point_x;\n    desired_relative_point_y = next_relative_desired_point_y;\nelse\n    desired_relative_point_x  = - 300;\n    desired_relative_point_y =  -250;\nend"("t"=w51, "index"=w78, "next_relative_desired_point_x"=w48, "next_relative_desired_point_y"=w47) -> ("desired_relative_point_x"=w46:dbl, "desired_relative_point_y"=w45:dbl, "index"=w79:dbl)  [unwired: 1 in, 1 out]
        "desired_relative_point_x" <- w46
        "desired_relative_point_y" <- w45
        n143 = feedback-in #1(w79) -> ()
        n144 = Subtract(x=w46, y=w50) -> (x-y=w159:ext)
        "error_relative_point_x" <- w159
        n145 = Subtract(x=w45, y=w49) -> (x-y=w144:ext)
        "error_relative_point_y" <- w144
        n146 = Build Array "创建数组"(w159, w144) -> (→"添加的数组":ext[])
        n147 = script code="load('F:\\capstone2025\\small_BP_rbf_DQN\\trained_net_color_2inputs_2outputs(2.1;1.3).mat', 'net');\npredicted_input  = [predicted_input_x; \n                               predicted_input_y];\npredicted_output = net(predicted_input);\npredicted_output_dr = predicted_output(1 , 1);\npredicted_output_pr = predicted_output(2 , 1);"("predicted_input_y"=w45, "predicted_input_x"=w46) -> ("predicted_output_dr"=w129:dbl, "predicted_output_pr"=w122:dbl)  [unwired: 1 in, 1 out]
        n148 = feedback-in #2(w144) -> ()
        n149 = Multiply(x=w159, y="Kp") -> (x*y=w166:ext)
        "Kp part" <- w166
        n150 = feedback-in #3(w159) -> ()
        n151 = Multiply(x=w144, y="Kp") -> (x*y=w152:ext)
        "Kp part" <- w152
        n152 = Subtract(x=w144, y=w151) -> (x-y=w149:ext)
        n153 = Subtract(x=w159, y=w165) -> (x-y=w163:ext)
        n154 = Multiply(x=w149, y="Kd") -> (x*y=w147:ext)
        "Kd part" <- w147
        n155 = Multiply(x=w163, y="Kd") -> (x*y=w161:ext)
        "Kd part" <- w161
        n156 = Insert Into Array(array=w146, new element=w144) -> (w145:dbl[])  [unwired: 1 in]
        n157 = feedback-in #4(w145) -> ()
        n158 = Insert Into Array(array=w160, new element=w159) -> (w158:dbl[])  [unwired: 1 in]
        n159 = feedback-in #5(w158) -> ()
        n160 = Add Array Elements(numeric array=w145) -> (sum=w142:dbl)
        n161 = Add Array Elements(numeric array=w158) -> (sum=w156:dbl)
        n162 = Multiply(x=w156, y="Ki") -> (x*y=w154:dbl)
        "Ki part" <- w154
        n163 = Multiply(x=w142, y="Ki") -> (x*y=w140:dbl)
        "Ki part" <- w140
        n164 = Bundle "捆绑"("cx"=w72, "cy"=w70) -> (w93:cluster{"cx":ext, "cy":ext})  [unwired: 1 in]
        n165 = Compound Arithmetic op=ADD(w152, w147, w140) -> (w61:ext)
        "u(t)_y" <- w61
        n166 = Compound Arithmetic op=ADD(w166, w161, w154) -> (w62:ext)
        "u(t)_x" <- w62
        n167 = Build Array (concatenate) "创建数组"(w84, w93) -> (w68:cluster{"cx":ext, "cy":ext}[])
        n168 = Multiply(x="K1", y=w61) -> (x*y=w44:ext)
        "delta_dr" <- w44
        n169 = Multiply(x="k2", y=w62) -> (x*y=w43:ext)
        "delta_pr" <- w43
        n170 = call "IMAQ Overlay Multiple Lines 2"("Image"=w81, "Line End Points"=w68, "Drawing Mode (Frame)"=w92, "Color"=u32 3071, "Width"=u32 5) -> ("Image Out"=→"彩色轨迹":T2)  [unwired: 9 in, 1 out]
        n171 = case shown="真" "打开彩色点轨迹" {
          tunnel: [_ w321] -> w67
          tunnel: w68 -> [_ w321]
          frame False {
          }
          frame True {
          }
        }
        n172 = feedback-in #6(w129) -> ()
        n173 = feedback-in #7(w122) -> ()
        n174 = Multiply(x=w122, y=0.95) -> (x*y=w118:dbl)
        n175 = Multiply(x=w129, y=0.95) -> (x*y=w125:dbl)
        n176 = Add(x=w118, y=w117) -> (x+y=w115:dbl)
        "MLP_pr" <- w115
        n177 = Add(x=w43, y=w115) -> (x+y=w113:ext)
        "magnet_input_pr" <- w113
        n178 = Add(x=w125, y=w124) -> (x+y=w116:dbl)
        "MLP_dr" <- w116
        n179 = Add(x=w44, y=w116) -> (x+y=w114:ext)
        "magnet_input_dr" <- w114
        n180 = case shown="\"Rotating Field\", 默认" "Parameter Settings" {
          tunnel: w318 -> [w334 w349 w364 w383 w402 w416 w434 w449]
          tunnel: w317 -> [w331 w348 w363 w382 w400 w415 w432 w448]
          tunnel: [w333 w347 w361 w381 w401 w414 w433 w447] -> w316
          tunnel: [w332 w346 w362 w380 w399 w413 w431 w446] -> w315
          tunnel: [w327 w340 w355 w376 w393 w408 w429 w441] -> w314
          tunnel: "Pause" -> [w325 w338 w353 w375 w392 w407 w424 w439]
          tunnel: [_ _ _ w372 _ _ _ _] -> w250
          tunnel: [_ _ _ w373 _ _ _ _] -> w248
          tunnel: w51 -> [_ _ _ w371 _ _ _ _]
          tunnel: [_ _ _ w370 _ _ _ _] -> w182
          tunnel: w114 -> [_ _ _ w369 _ _ _ _]
          tunnel: w113 -> [_ _ _ w368 _ _ _ _]
          frame "Gradient Field " {
            n181 = case shown="假" w325 {
              tunnel: ["Ag" 0.0] -> w326
              frame False {
              }
              frame True {
              }
            }
            n182 = Build Array(1.0, w326, "pg", "dg", "fg") -> (w327:dbl[])
            n183 = shared-variable-write(w334, w331, w327, 1000 ("timeout ms (-1)")) -> (w333:refnum<k21>, w332:errorcluster)  [unwired: 1 out]
          }
          frame "Oscillating Field" {
            n184 = case shown="假" w338 {
              tunnel: ["AoOF" 0.0] -> w339
              frame False {
              }
              frame True {
              }
            }
            n185 = Build Array(2.0, w339, "oo", "fo", "po", "do") -> (w340:dbl[])
            n186 = shared-variable-write(w349, w348, w340, 1000 ("timeout ms (-1)")) -> (w347:refnum<k21>, w346:errorcluster)  [unwired: 1 out]
          }
          frame "Conical Field" {
            # "FG"
            n187 = case shown="假" w353 {
              tunnel: ["Ac" 0.0] -> w354
              frame False {
              }
              frame True {
              }
            }
            n188 = Build Array(3.0, w354, "wc", "pc", "dc", "cc") -> (w355:dbl[])
            n189 = shared-variable-write(w364, w363, w355, 1000 ("timeout ms (-1)")) -> (w361:refnum<k21>, w362:errorcluster)  [unwired: 1 out]
          }
          frame "Rotating Field", Default {
            n190 = case shown="假" w375 {
              tunnel: ["Ar" 0.0] -> w372
              frame False {
              }
              frame True {
              }
            }
            n191 = case shown="真" "磁场变换" {
              tunnel: [sgl 0.0 ("pr") w387] -> w378
              tunnel: [sgl 0.0 ("dr") w388] -> w373
              tunnel: w371 -> [_ w389]
              tunnel: [_ w387] -> w370
              tunnel: w369 -> [_ w388]
              tunnel: w368 -> [_ w387]
              frame False {
              }
              frame True {
                n192 = formula code="int p;\n    int q;\n    q = t/50 ;  \n    p = q%36; //用来构造循环\n    dr = -180 + (p*10);\n\n    int p2;\n    int q2;\n    q2 = q/(72);\n    p2 = q2%36; //用来构造循环\n    pr =  -40 + p2*10;"("t"=w389) -> ()  [unwired: 2 out]
                "dr" <- w388
                "pr" <- w387
              }
            }
            n193 = Build Array(4.0, w372, "wr", w378, w373) -> (w376:ext[])
            n194 = shared-variable-write "向流中写入单个元素"(w383, w382, w376, 1000 ("timeout ms (-1)")) -> (w381:refnum<k21>, w380:errorcluster)  [unwired: 1 out]
          }
          frame "Disassembly" {
            n195 = case shown="假" w392 {
              tunnel: ["Dis strength(mT)" 0.0] -> w397
              frame False {
              }
              frame True {
              }
            }
            n196 = Build Array(5.0, w397, "Dis tumbling frequency (Hz)", "Dis phase frequency (Hz)", "Dis phase step") -> (w393:dbl[])
            n197 = shared-variable-write(w402, w400, w393, 1000 ("timeout ms (-1)")) -> (w401:refnum<k21>, w399:errorcluster)  [unwired: 1 out]
          }
          frame "Swarm" {
            n198 = case shown="假" w407 {
              tunnel: ["Swa strength (mT)" 0.0] -> w406
              frame False {
              }
              frame True {
              }
            }
            n199 = Build Array(6.0, w406, "Swa frequency (Hz)", "Swa pitch angle (deg)", "Swa direction angle (deg)", "Swa ratio") -> (w408:dbl[])
            n200 = shared-variable-write(w416, w415, w408, 1000 ("timeout ms (-1)")) -> (w414:refnum<k21>, w413:errorcluster)  [unwired: 1 out]
          }
          frame "Ribbon Oscillating Field" {
            n201 = case shown="假" w424 {
              tunnel: ["Strength (mT)" 0.0] -> w423
              frame False {
              }
              frame True {
              }
            }
            n202 = Build Array(7.0, w423, "Frequency (Hz)", "Ratio (A/C)", "Direction Angle (deg)", "Pitch Angle (rotating around Origin, deg)", "Pitch Angle (rotating around Constant, deg)") -> (w429:dbl[])
            n203 = shared-variable-write(w434, w432, w429, 1000 ("timeout ms (-1)")) -> (w433:refnum<k21>, w431:errorcluster)  [unwired: 1 out]
          }
          frame "Elliptical Field" {
            n204 = case shown="假" w439 {
              tunnel: ["Ar 2" 0.0] -> w440
              frame False {
              }
              frame True {
              }
            }
            n205 = Build Array(8.0, w440, "wr  2", "pr  2", "dr  2", "ratio", "p_x") -> (w441:dbl[])
            n206 = shared-variable-write(w449, w448, w441, 1000 ("timeout ms (-1)")) -> (w447:refnum<k21>, w446:errorcluster)  [unwired: 1 out]
          }
        }
        "Array" <- w314
        "场强" <- w250
        "dr" <- w248
        n207 = Build Array (concatenate)(w247, w248) -> (w244:ext[])
        "direction angle" <- w244
        n208 = Build Array (concatenate)(w181, w182) -> (w180:ext[])
        n209 = Build Array (concatenate)(w249, w250) -> (w245:dbl[])
        "strength" <- w245
        n210 = Or(x=w315, y="Stop") -> (x .or. y?=w311:bool)
        n211 = Build Array(w246, w245, w244, w243, w238, w242, w241, w240, w234, w230, w211, w210, w197, w193, w188, w180) -> (→"all parameters":ext[][])
        "Numeric 5" <- w51
        "T" <- w51
        "T" <- w51
        "prev_end_point_x" <- w226
        "prev_end_point_y" <- w222
        "prev time" <- w205
      }
    }
    frame #3 {
      # "4. The error -314220 indicates that the other endpoint has been destroyed. The VI ignores this error."
      # "3. Destroy the stream endpoint when you click Stop or when an error occurs."
      # "Close"
      n212 = Flush Stream(8:w459, 11:w462) -> (0:w460:errorcluster, 3:w461:refnum<k21>)  [unwired: 2 in, 1 out]
      n213 = Destroy Stream Endpoint(8:w460, 11:w461) -> (0:w454:errorcluster)
      n214 = Unbundle By Name(w454) -> ("code"=w458:i32)
      n215 = xnode "Error Ring"() -> ("错误输出"=w455:errorcluster)
      n216 = Not Equal?(x=w458, y=-314220) -> (x != y?=w456:bool)
      n217 = Select(t=w454, s=w456, f=w455) -> (s? t:f=→"error out":errorcluster)
    }
  }
